vi "get_proc_andIDs.vi"() -> (0 "return":i32, 1 "procese":string[](array[string]), 2 "IDs 2":u32[](array[numeric]))   [LabVIEW 2016]
uses:
  processHandles.dll
panel:
  in  "procs 3":u16[](array[numeric])=array[5001 elements]
  out "procs":u16[](array[numeric])
  in  "IDs":u32[](array[numeric])=array[5001 elements]
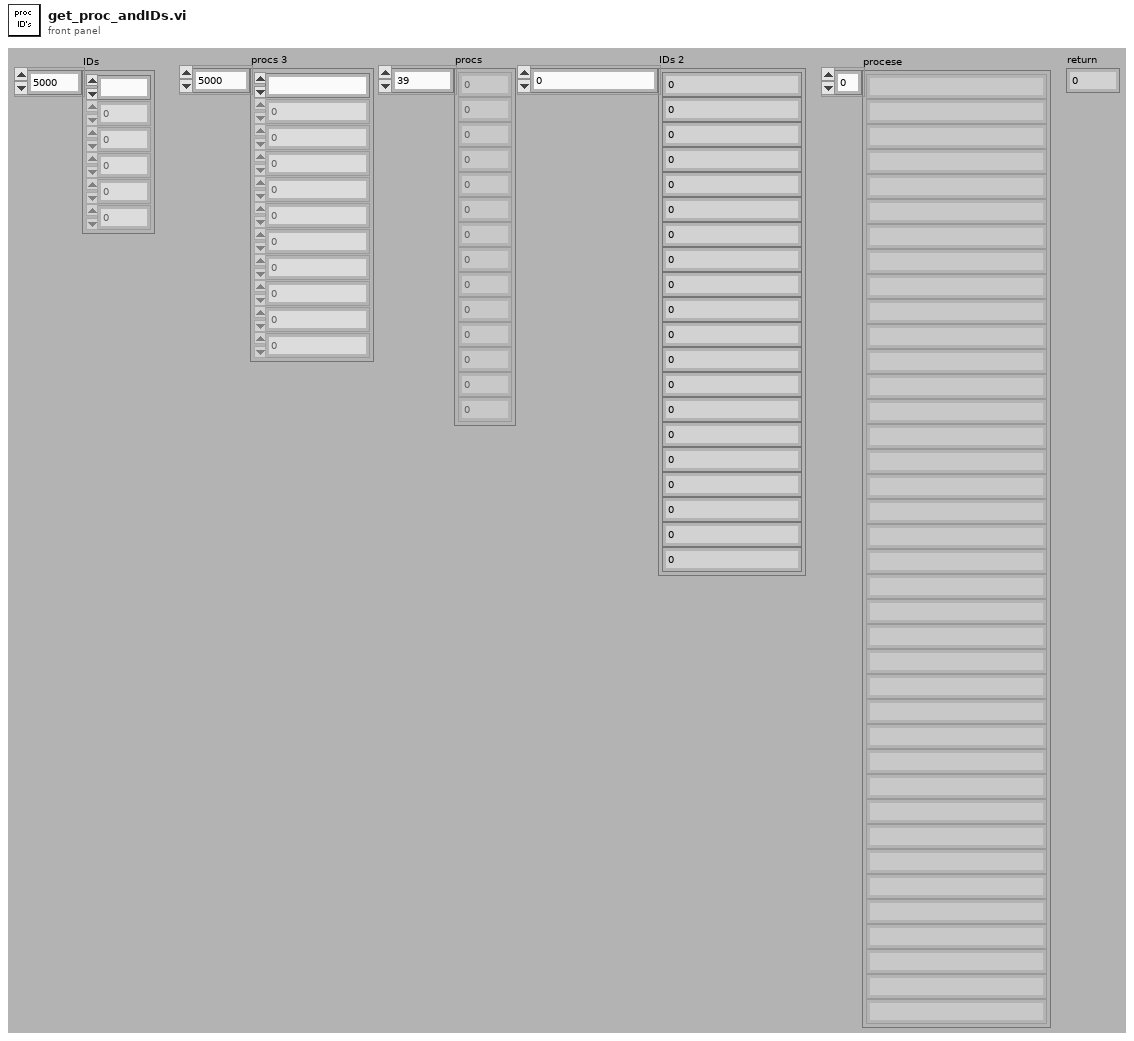
[diagram p1: front panel]
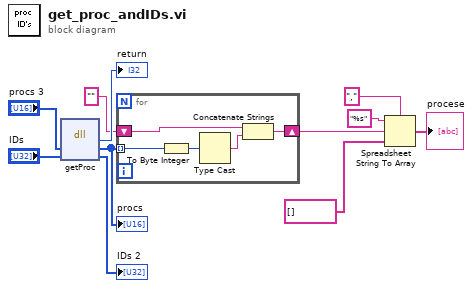
[diagram p0: block diagram]
diagram:
  n1 = dll-call lib="C:/Technology Lab/NI-2010/Trunk/Utility/Project Memory Manager/Project Manager/processHandles.dll" fn="getProc"("procs"="procs 3", "IDs"="IDs") -> ("return type"=→"return":i32, "procs"=w7:u16[], "IDs"=→"IDs 2":u32[])  [unwired: 3 in, 2 out]
  "procs" <- w7
  n2 = for {
    tunnel: w7 -> [w13] mode=indexing
    shift-right: [w14] -> w6
    shift-left: "" -> [w16]
    n3 = To Byte Integer(number=w13) -> (8bit integer=w12:i8)
    n4 = Type Cast(x=w12) -> (*(type *) &x=w15:string)  [unwired: 1 out]
    n5 = Concatenate Strings(w16, w15) -> (w14:string)
  }
  n6 = Spreadsheet String To Array(delimiter (Tab)=",", format string="%s", spreadsheet string=w6, array type (2D Dbl)=string[] []) -> (array=→"procese":string[])
